vi "Cumulative Function Computation.vi"(6 "Normalized (F)":bool, 8 "Error In":errorcluster, 11 "Array":dbl[](array[numeric])) -> (0 "Error Out":errorcluster, 3 "Cumulative Function Array":dbl[](array[numeric]))   [LabVIEW 2021, in "Arrays.lvlib"]
doc: "Extract IRF from provided decay and time constant"
uses:
  Arrays.lvlib
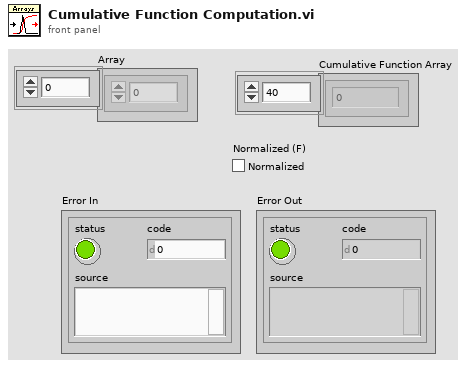
[diagram p1: front panel]
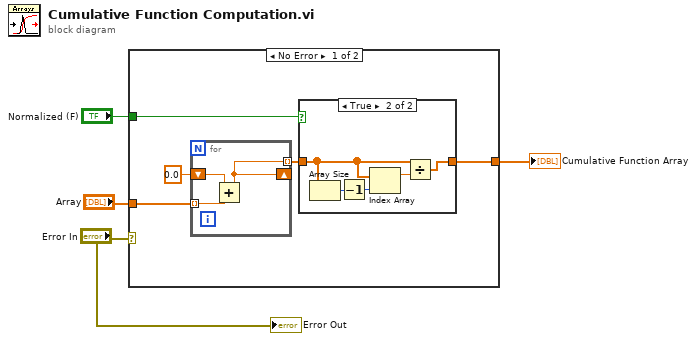
[diagram p0: block diagram]
diagram:
  n1 = case shown="No Error" "Error In" {
    tunnel: "Array" -> [w9 _]
    tunnel: "Normalized (F)" -> [w6 _]
    tunnel: [w5 _] -> w2
    frame No Error {
      n2 = for {
        tunnel: w9 -> [w17] mode=indexing
        shift-right: [w16] -> _
        shift-left: 0.0 -> [w18]
        tunnel: [w16] -> w7 mode=indexing
        n3 = Add(x=w18, y=w17) -> (x+y=w16:dbl)
      }
      n4 = case shown="True" w6 {
        tunnel: w7 -> [w10 w13]
        tunnel: [w10 w14] -> w5
        frame False {
        }
        frame True {
          n5 = Array Size(array=w13) -> (size(s)=w12:i32)
          n6 = Decrement(x=w12) -> (x-1=w11:i32)
          n7 = Index Array(array=w13, index=w11) -> (element=w15:dbl)
          n8 = Divide(x=w13, y=w15) -> (x/y=w14:dbl[])
        }
      }
    }
    frame Error {
    }
  }
  "Cumulative Function Array" <- w2
  "Error Out" <- "Error In"
